vi "Rectangle ComparisonPegPYLB.vi"(6 "Line Border":cluster{"Top":dbl, "Bottom":dbl}={"Top"=6.0, "Bottom"=1.0}, 9 "Second":dbl[](array[numeric]), 11 "First":dbl[](array[numeric])) -> (0 "Rect":T1, 1 "Line":T1, 3 "Scores":T2)   [LabVIEW 2016]
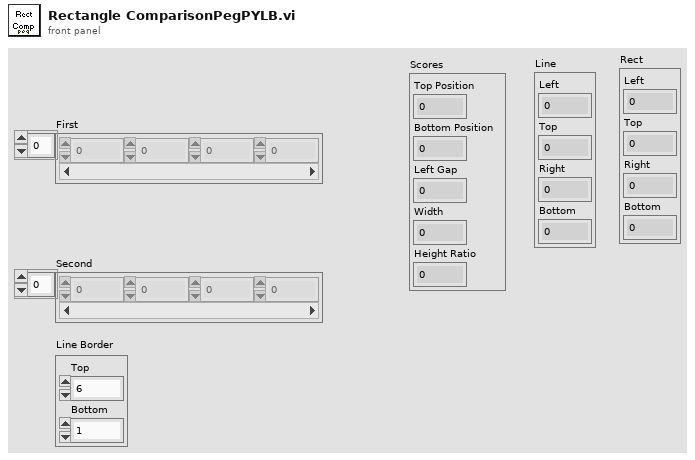
[diagram p1: front panel]
types:
  T1 = cluster{"Left":dbl, "Top":dbl, "Right":dbl, "Bottom":dbl}
  T2 = cluster{"Top Position":dbl, "Bottom Position":dbl, "Left Gap":dbl, "Width":dbl, "Height Ratio":dbl}
  T3 = cluster{"[0]":dbl, "[1]":dbl, "[2]":dbl, "[3]":dbl}
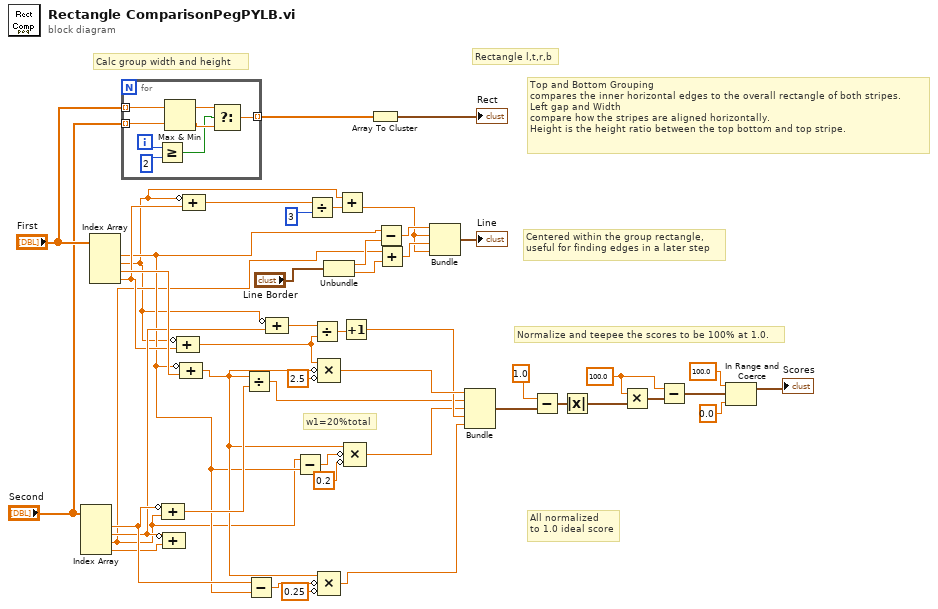
[diagram p0: block diagram]
diagram:
  w32 = 100.0 ("x/y")
  # "w1=20%total"
  # "Centered within the group rectangle,\nuseful for finding edges in a later step"
  # "All normalized\nto 1.0 ideal score"
  # "Normalize and teepee the scores to be 100% at 1.0."
  # "Top and Bottom Grouping\ncompares the inner horizontal edges to the overall rectangle of both stripes.\nLeft gap and Width\ncompare how the stripes are aligned horizontally.\nHeight is the height ratio between the top bottom and top stripe."
  # "Calc group width and height"
  # "Rectangle l,t,r,b"
  n1 = Index Array(array="Second") -> (element #1=w47:dbl, element #2=w23:dbl, element #3=w5:dbl, element #4=w24:dbl)  [unwired: 4 in]
  n2 = Index Array(array="First") -> (element #1=w6:dbl, element #2=w1:dbl, element #3=w43:dbl, element #4=w7:dbl)  [unwired: 4 in]
  n3 = for {
    tunnel: "First" -> [w55] mode=indexing
    tunnel: "Second" -> [w54] mode=indexing
    tunnel: [w48] -> w37 mode=indexing
    i -> [w52]
    n4 = Greater Or Equal?(x=w52, y=2) -> (x >= y?=w49:bool)
    n5 = Max & Min(x=w55, y=w54) -> (max(x,y)=w51:dbl, min(x,y)=w50:dbl)
    n6 = Select(t=w51, s=w49, f=w50) -> (s? t:f=w48:dbl)
  }
  n7 = Compound Arithmetic op=ADD(invert w47, w5) -> (w18:dbl)
  n8 = Compound Arithmetic op=ADD(invert w23, w24) -> ()  [unwired: 1 out]
  n9 = Compound Arithmetic op=ADD(invert w1, w7) -> (w14:dbl)
  n10 = Compound Arithmetic op=ADD(invert w6, w43) -> (w10:dbl)
  n11 = Compound Arithmetic op=ADD(invert w1, w7) -> (w42:dbl)
  n12 = Divide(x=w10, y=w18) -> (x/y=w22:dbl)
  n13 = Subtract(x=w47, y=w6) -> (x-y=w12:dbl)
  n14 = Compound Arithmetic op=ADD(invert w1, w23) -> (w15:dbl)
  n15 = Subtract(x=w5, y=w6) -> (x-y=w17:dbl)
  n16 = Divide(x=w42, y=3) -> (x/y=w8:dbl)
  n17 = Divide(x=w15, y=w14) -> (x/y=w13:dbl)
  n18 = Compound Arithmetic op=MULTIPLY(w14, invert w10, invert 2.5 ("value")) -> (w46:dbl)
  n19 = Compound Arithmetic op=MULTIPLY(w10, invert w12, invert 0.25 ("value")) -> (w44:dbl)
  n20 = Unbundle("Line Border") -> ("Top"=w19:dbl, "Bottom"=w20:dbl)
  n21 = Add(x=w1, y=w8) -> (x+y=w2:dbl)
  n22 = Increment(x=w13) -> (x+1=w45:dbl)
  n23 = Compound Arithmetic op=MULTIPLY(w10, invert w17, invert 0.2 ("value")) -> (w35:dbl)
  n24 = Array To Cluster(array=w37) -> (cluster=→"Rect":T3)
  n25 = Subtract(x=w6, y=w19) -> (x-y=w3:dbl)
  n26 = Add(x=w5, y=w20) -> (x+y=w4:dbl)
  n27 = Bundle(w3, w2, w4, w2) -> (→"Line":cluster{dbl, dbl, dbl, dbl})  [unwired: 1 in]
  n28 = Bundle(w46, w22, w35, w45, w44) -> (w26:cluster{dbl, dbl, dbl, dbl, dbl})  [unwired: 1 in]
  n29 = Subtract(x=1.0 ("y"), y=w26) -> (x-y=w30:cluster{dbl, dbl, dbl, dbl, dbl})
  n30 = Absolute Value(x=w30) -> (abs(x)=w33:cluster{dbl, dbl, dbl, dbl, dbl})
  n31 = Multiply(x=w32, y=w33) -> (x*y=w34:cluster{dbl, dbl, dbl, dbl, dbl})
  n32 = Subtract(x=w32, y=w34) -> (x-y=w29:cluster{dbl, dbl, dbl, dbl, dbl})
  n33 = In Range and Coerce(upper limit=100.0, x=w29, lower limit=0.0) -> (coerced(x)=→"Scores":cluster{dbl, dbl, dbl, dbl, dbl})  [unwired: 1 out]
